vi "Call Inspect.vi"(4 "Msg":refnum<class "Msg.lvclass">, 6 "Within Unified Msgs":bool, 7 "Actor in":refnum<class "Actor.lvclass">, 8 "Error in":errorcluster) -> (0 "Error out":errorcluster, 2 "Proceed":bool=TRUE, 5 "Actor out":refnum<class "Actor.lvclass">)   [LabVIEW 2025, in "jettl.lvlib"]
uses:
  jettl.lvlib
  Msg/Msg.lvclass
  Actor/Actor.lvclass
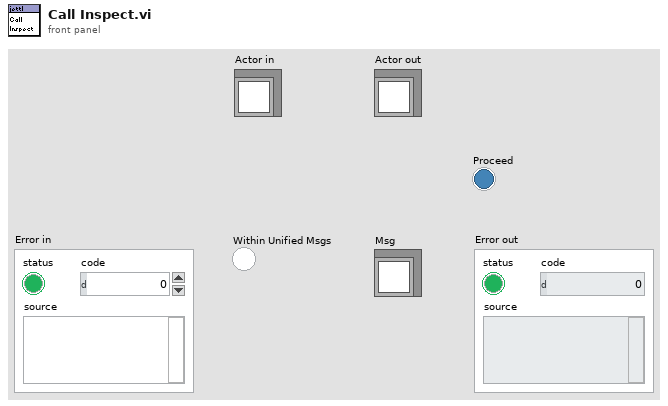
[diagram p1: front panel]
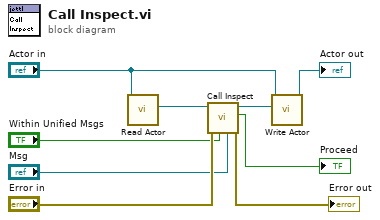
[diagram p0: block diagram]
diagram:
  n1 = call-dynamic "Read Actor.vi"("Actor in"="Actor in") -> ("Actor"=w9:refnum<class "Actor.lvclass">)  [unwired: 10 in]
  n2 = call-dynamic "Call Inspect.vi"("Msg"="Msg", "Within Unified Msgs"="Within Unified Msgs", "Error in"="Error in", "Actor in"=w9) -> ("Error out"=→"Error out":errorcluster, "Proceed"=→"Proceed":bool, "Actor out"=w8:refnum<class "Actor.lvclass">)  [unwired: 5 in]
  n3 = call-dynamic "Write Actor.vi"("Actor"=w8, "Actor in"="Actor in") -> ("Actor out"=→"Actor out":refnum<class "Actor.lvclass">)  [unwired: 9 in]
